vi "MeasureDarkCurrent.vi"(8 "Multimeter GPIB Address":string, 9 "Amplifier":refnum<visa-resource-name>) -> (0 "Amplifier Error":errorcluster, 1 "Amplifier Settings":T1)   [LabVIEW 2017]
uses:
  AmplifierSettings.ctl
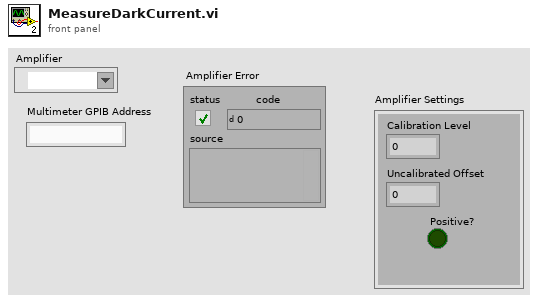
[diagram p1: front panel]
types:
  T1 = typedef "AmplifierSettings.ctl" = cluster{"Calibration Level":dbl, "Uncalibrated Offset":dbl, "Positive?":bool}
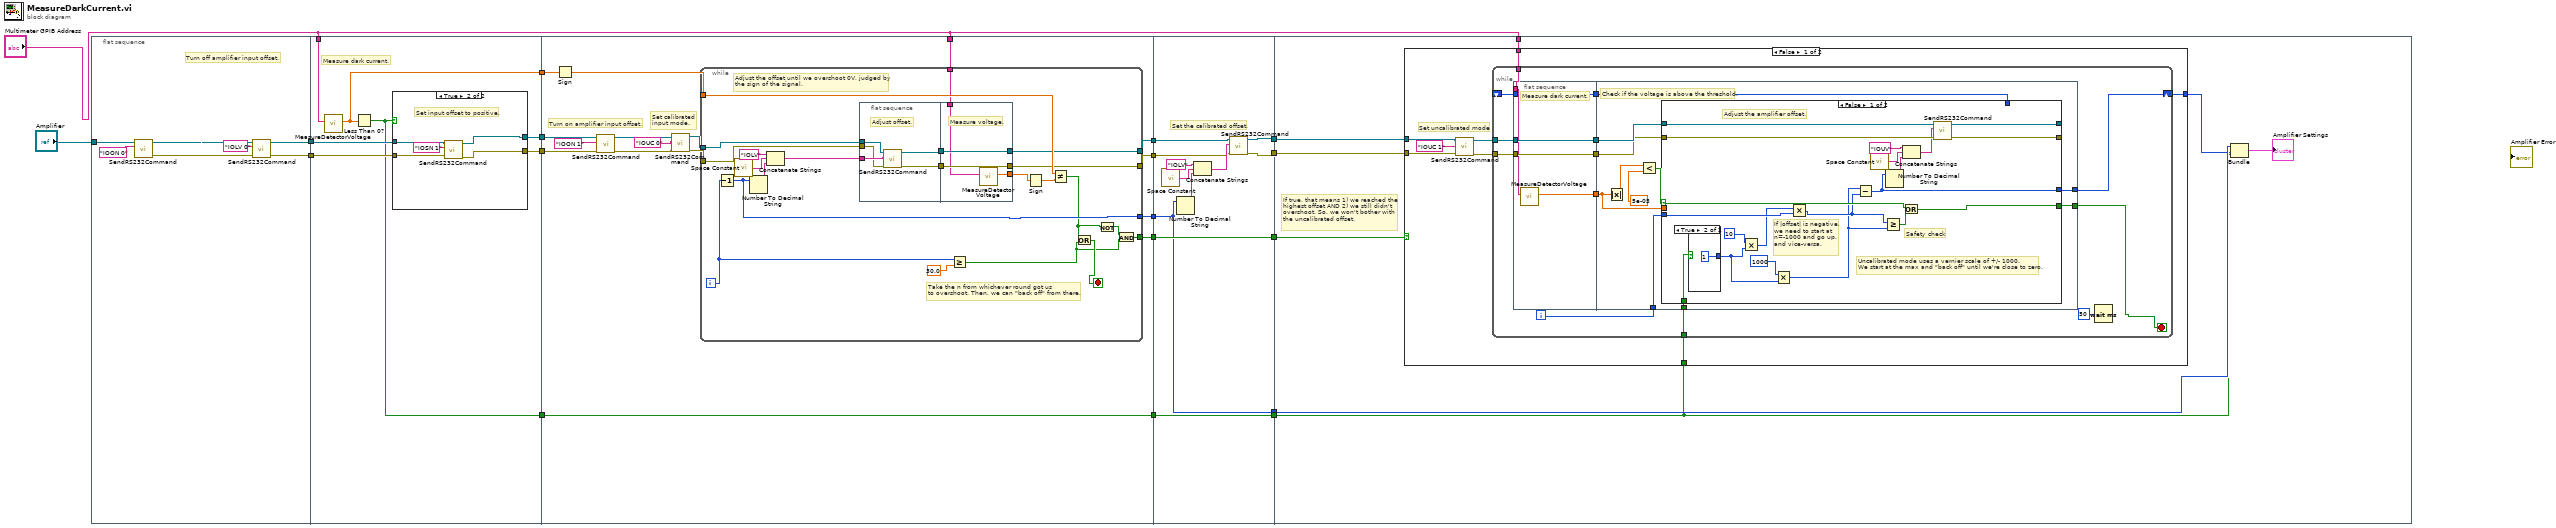
[diagram p0: block diagram]
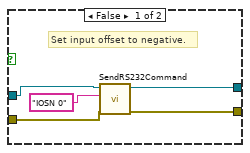
[diagram p2: hidden frame]
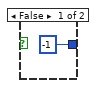
[diagram p3: hidden frame]
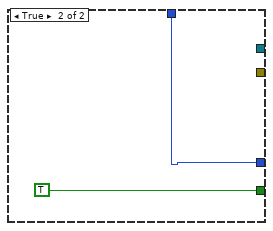
[diagram p4: hidden frame]
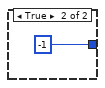
[diagram p5: hidden frame]
diagram:
  n1 = flat-sequence {
    tunnel: "Amplifier" -> [w25]
    tunnel: [w23] -> w17
    tunnel: [w22] -> w16
    tunnel: w17 -> [w32]
    tunnel: w16 -> [w31]
    tunnel: [w30] -> w15
    tunnel: [w29] -> w14
    tunnel: [w28] -> w13
    tunnel: "Multimeter GPIB Address" -> [w27]
    tunnel: [w26] -> w1
    tunnel: w15 -> [w57]
    tunnel: w14 -> [w56]
    tunnel: w13 -> [w55]
    tunnel: [w53] -> w12
    tunnel: [w52] -> w11
    tunnel: [w51] -> w10
    tunnel: [w45] -> w6
    tunnel: "Multimeter GPIB Address" -> [w44]
    tunnel: [w43] -> w2
    tunnel: w1 -> [w43]
    tunnel: w12 -> [w95]
    tunnel: w11 -> [w96]
    tunnel: w10 -> [w91]
    tunnel: [w94] -> w9
    tunnel: [w93] -> w8
    tunnel: [w92] -> w7
    tunnel: w6 -> [w92]
    tunnel: [w91] -> w4
    tunnel: [w90] -> w3
    tunnel: w2 -> [w90]
    tunnel: w9 -> [w107]
    tunnel: w8 -> [w108]
    tunnel: w7 -> [w106]
    tunnel: "Multimeter GPIB Address" -> [w105]
    tunnel: w4 -> [w104]
    tunnel: w3 -> [w101]
    frame #0 {
      # "Turn off amplifier input offset."
      n2 = call "SendRS232Command.vi"("Command"="IOON 0", "VISA/RS232 Device In"=w25) -> ("error out"=w20:errorcluster, "VISA/RS232 Device Out"=w21:refnum<visa-resource-name>)  [unwired: 8 in]
      n3 = call "SendRS232Command.vi"("error in (no error)"=w20, "Command"="IOLV 0", "VISA/RS232 Device In"=w21) -> ("error out"=w22:errorcluster, "VISA/RS232 Device Out"=w23:refnum<visa-resource-name>)  [unwired: 7 in]
    }
    frame #1 {
      # "Measure dark current."
      n4 = call "MeasureDetectorVoltage.vi"("GPIB Address"=w27) -> ("Average Voltage"=w28:dbl)  [unwired: 10 in]
      n5 = Less Than 0?(x=w28) -> (x < 0?=w26:bool)
      n6 = case shown="True" w26 {
        tunnel: w32 -> [w36 w42]
        tunnel: w31 -> [w35 w41]
        tunnel: [w34 w39] -> w30
        tunnel: [w33 w38] -> w29
        frame False {
          # "Set input offset to negative."
          n7 = call "SendRS232Command.vi"("error in (no error)"=w35, "Command"="IOSN 0", "VISA/RS232 Device In"=w36) -> ("error out"=w33:errorcluster, "VISA/RS232 Device Out"=w34:refnum<visa-resource-name>)  [unwired: 7 in]
        }
        frame True {
          # "Set input offset to positive."
          n8 = call "SendRS232Command.vi"("error in (no error)"=w41, "Command"="IOSN 1", "VISA/RS232 Device In"=w42) -> ("error out"=w38:errorcluster, "VISA/RS232 Device Out"=w39:refnum<visa-resource-name>)  [unwired: 7 in]
        }
      }
    }
    frame #2 {
      # "Set calibrated \ninput mode."
      # "Turn on amplifier input offset."
      n9 = Sign(1:w55) -> (0:w54:dbl)
      n10 = call "SendRS232Command.vi"("error in (no error)"=w56, "Command"="IOON 1", "VISA/RS232 Device In"=w57) -> ("error out"=w48:errorcluster, "VISA/RS232 Device Out"=w49:refnum<visa-resource-name>)  [unwired: 7 in]
      n11 = call "SendRS232Command.vi"("error in (no error)"=w48, "Command"="IOUC 0", "VISA/RS232 Device In"=w49) -> ("error out"=w46:errorcluster, "VISA/RS232 Device Out"=w47:refnum<visa-resource-name>)  [unwired: 7 in]
      n12 = while {
        tunnel: w47 -> [w76]
        tunnel: w46 -> [w75]
        tunnel: w54 -> [w71]
        tunnel: [w65] -> w51
        tunnel: [w67] -> w53
        tunnel: [w66] -> w52
        tunnel: [w60] -> w45
        tunnel: w44 -> [w59]
        i -> [w73]
        stop <- w64 stop-if-true
        # "Take the n from whichever round got us \nto overshoot. Then, we can \"back off\" from there."
        # "Adjust the offset until we overshoot 0V, judged by\nthe sign of the signal."
        n13 = Decrement(x=w73) -> (x-1=w65:i32)
        n14 = call <vilib>:"Space Constant.vi"() -> ("String"=w79:string)
        n15 = Number To Decimal String(number=w65) -> (decimal integer string=w78:string)  [unwired: 1 in]
        n16 = Concatenate Strings("IOLV", w79, w78) -> (w77:string)
        n17 = flat-sequence {
          tunnel: w77 -> [w85]
          tunnel: w76 -> [w84]
          tunnel: w75 -> [w83]
          tunnel: [w82] -> w70
          tunnel: [w81] -> w69
          tunnel: [w89] -> w68
          tunnel: w70 -> [w88]
          tunnel: w69 -> [w87]
          tunnel: [w88] -> w67
          tunnel: [w87] -> w66
          tunnel: w59 -> [w86]
          frame #0 {
            # "Adjust offset."
            n18 = call "SendRS232Command.vi"("error in (no error)"=w83, "Command"=w85, "VISA/RS232 Device In"=w84) -> ("error out"=w81:errorcluster, "VISA/RS232 Device Out"=w82:refnum<visa-resource-name>)  [unwired: 7 in]
          }
          frame #1 {
            # "Measure voltage."
            n19 = call "MeasureDetectorVoltage.vi"("GPIB Address"=w86) -> ("Average Voltage"=w89:dbl)  [unwired: 10 in]
          }
        }
        n20 = Greater Or Equal?(x=w73, y=30.0) -> (x >= y?=w61:bool)
        n21 = Sign(1:w68) -> (0:w72:dbl)
        n22 = Not Equal?(x=w71, y=w72) -> (x != y?=w63:bool)
        n23 = Or(x=w63, y=w61) -> (x .or. y?=w64:bool)
        n24 = Not(x=w63) -> (.not. x?=w62:bool)
        n25 = And(x=w62, y=w61) -> (x .and. y?=w60:bool)
      }
    }
    frame #3 {
      # "Set the calibrated offset."
      n26 = call <vilib>:"Space Constant.vi"() -> ("String"=w99:string)
      n27 = Number To Decimal String(number=w91) -> (decimal integer string=w100:string)  [unwired: 1 in]
      n28 = Concatenate Strings("IOLV", w99, w100) -> (w97:string)
      n29 = call "SendRS232Command.vi"("error in (no error)"=w96, "Command"=w97, "VISA/RS232 Device In"=w95) -> ("error out"=w94:errorcluster, "VISA/RS232 Device Out"=w93:refnum<visa-resource-name>)  [unwired: 7 in]
    }
    frame #4 {
      # "If true, that means 1) we reached the \nhighest offset AND 2) we still didn't \novershoot. So, we won't bother with \nthe uncalibrated offset."
      n30 = case shown="False" w106 {
        tunnel: w108 -> [w113 _]
        tunnel: w107 -> [w112 _]
        tunnel: w105 -> [w111 _]
        tunnel: [w110 -1] -> w103
        tunnel: w101 -> [w109 _]
        frame False {
          # "Set uncalibrated mode"
          n31 = call "SendRS232Command.vi"("error in (no error)"=w112, "Command"="IOUC 1", "VISA/RS232 Device In"=w113) -> ("error out"=w115:errorcluster, "VISA/RS232 Device Out"=w116:refnum<visa-resource-name>)  [unwired: 7 in]
          n32 = while {
            tunnel: w116 -> [w127]
            tunnel: w115 -> [w125]
            tunnel: w111 -> [w121]
            shift-right: [w120] -> w110
            shift-left: _ -> [w118]
            tunnel: w109 -> [w117]
            i -> [w124]
            stop <- w123 stop-if-true
            n33 = flat-sequence {
              tunnel: [w134] -> w129
              tunnel: [w133] -> w128
              tunnel: w127 -> [w133]
              tunnel: [w132] -> w126
              tunnel: w125 -> [w132]
              tunnel: w121 -> [w131]
              tunnel: [w130] -> w119
              tunnel: w118 -> [w130]
              tunnel: w129 -> [w142]
              tunnel: [w141] -> w123
              tunnel: w128 -> [w140]
              tunnel: w126 -> [w139]
              tunnel: w124 -> [w138]
              tunnel: [w137] -> w120
              tunnel: w119 -> [w136]
              tunnel: w117 -> [w135]
              frame #0 {
                # "Measure dark current."
                n34 = call "MeasureDetectorVoltage.vi"("GPIB Address"=w131) -> ("Average Voltage"=w134:dbl)  [unwired: 10 in]
              }
              frame #1 {
                # "Check if the voltage is above the threshold."
                n35 = Absolute Value(x=w142) -> (abs(x)=w145:dbl)
                n36 = Less?(x=w145, y=5e-05) -> (x < y?=w143:bool)
                n37 = case shown="False" w143 {
                  selector: w143 -> [w156 _]
                  tunnel: w142 -> [_ _]
                  tunnel: [w157 TRUE] -> w141
                  tunnel: w140 -> [w165 _]
                  tunnel: w139 -> [w164 _]
                  tunnel: w138 -> [w154 _]
                  tunnel: [w159 _] -> _
                  tunnel: [w158 _] -> _
                  tunnel: [w152 w168] -> w137
                  tunnel: w136 -> [_ w168]
                  tunnel: w135 -> [w151 _]
                  frame False {
                    # "If |offset| is negative,\nwe need to start at \nn=-1000 and go up, \nand vice-versa."
                    # "Safety check"
                    # "Uncalibrated mode uses a vernier scale of +/- 1000. \nWe start at the max and \"back off\" until we're close to zero."
                    # "Adjust the amplifier offset."
                    n38 = case shown="True" w151 {
                      tunnel: [-1 1] -> w148
                      frame False {
                      }
                      frame True {
                      }
                    }
                    n39 = Multiply(x=10, y=w148) -> (x*y=w149:i32)
                    n40 = Multiply(x=1000, y=w148) -> (x*y=w146:i32)
                    n41 = Multiply(x=w149, y=w154) -> (x*y=w153:i32)
                    n42 = Subtract(x=w146, y=w153) -> (x-y=w152:i32)
                    n43 = call <vilib>:"Space Constant.vi"() -> ("String"=w162:string)
                    n44 = Greater Or Equal?(x=w153, y=w146) -> (x >= y?=w155:bool)
                    n45 = Number To Decimal String(number=w152) -> (decimal integer string=w161:string)  [unwired: 1 in]
                    n46 = Concatenate Strings("IOUV", w162, w161) -> (w160:string)
                    n47 = Or(x=w156, y=w155) -> (x .or. y?=w157:bool)
                    n48 = call "SendRS232Command.vi"("error in (no error)"=w164, "Command"=w160, "VISA/RS232 Device In"=w165) -> ("error out"=w158:errorcluster, "VISA/RS232 Device Out"=w159:refnum<visa-resource-name>)  [unwired: 7 in]
                  }
                  frame True {
                  }
                }
              }
            }
            n49 = Wait (ms)(milliseconds to wait=u32 50) -> ()  [unwired: 1 out]
          }
        }
        frame True {
        }
      }
      n50 = Bundle(w104, w103, w101) -> (→"Amplifier Settings":cluster{i32, i32, bool})  [unwired: 1 in]
    }
  }
